vi "SLSC Separate Channels.vi"(8 "error in (no error)":errorcluster, 11 "Item Refs In":T1[](array[typedef]) format="%.0x") -> (0 "error out":errorcluster, 1 "Not Channels":T1[](array[typedef]) format="%.0x", 2 "Output Channels":T1[](array[typedef]) format="%.0x", 3 "Input Channels":T1[](array[typedef]) format="%.0x")   [LabVIEW 2020, in "SLSC EDS System Explorer.lvlib"]
uses:
  SLSC EDS System Explorer.lvlib
  <vilib>/NI VeriStand/Custom Device API/Custom Device Item Ref.ctl
  <vilib>/NI VeriStand/Custom Device API/Custom Device Channel Type.ctl
  <vilib>/NI VeriStand/Custom Device API/Custom Device API.lvlib
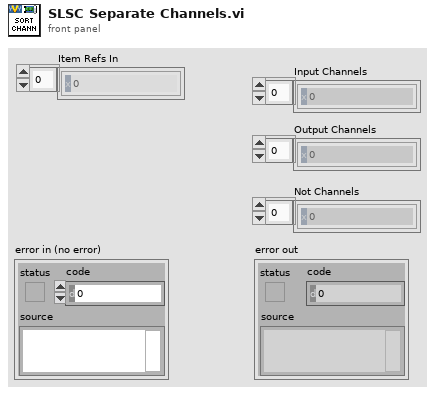
[diagram p1: front panel]
types:
  T1 = typedef "Custom Device API.lvlib/Custom Device Item Ref.ctl" = u64
  T2 = typedef "Custom Device API.lvlib/Custom Device Channel Type.ctl" = enum16{"Input", "Output"}
  T3 = typedef "Custom Device API.lvlib/Custom Device Channel.ctl" = cluster{"Type":T2, "Units":string, "Default Value":dbl, "Faultable":bool, "Scalable":bool}
  T4 = typedef "Custom Device API.lvlib/Custom Device Item Info.ctl" = cluster{"Name":string, "Is Channel":bool, "GUID":string, "Is Waveform":bool}
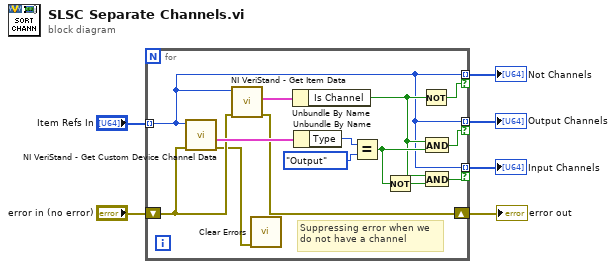
[diagram p0: block diagram]
diagram:
  n1 = for {
    tunnel: "Item Refs In" -> [w9] mode=indexing
    tunnel: [w9] -> w4 mode=indexing if=w13
    tunnel: [w9] -> w5 mode=indexing if=w14
    tunnel: [w9] -> w6 mode=indexing if=w11
    shift-right: [w10] -> w1
    shift-left: "error in (no error)" -> [w8]
    # "Suppressing error when we\ndo not have a channel"
    n2 = call <vilib>:"NI VeriStand - Get Custom Device Channel Data.vi"("error in (no error)"=w8, "Channel Ref in"=w9) -> ("error out"=w7:errorcluster, "Channel"=w20:T3)  [unwired: 4 in, 4 out]
    n3 = call <vilib>:"NI VeriStand - Get Item Data.vi"("error in (no error)"=w8, "Item Ref in"=w9) -> ("error out"=w10:errorcluster, "Item Info"=w19:T4)  [unwired: 6 in, 2 out]
    n4 = call <vilib>:"Clear Errors.vi"("error in (no error)"=w7) -> ()  [unwired: 5 in, 2 out]
    n5 = Unbundle By Name(w19) -> ("Is Channel"=w12:bool)
    n6 = Unbundle By Name(w20) -> ("Type"=w17:T2)
    n7 = Equal?(x=w17, y=Custom_Device_Channel_Type."Output" ("Type")) -> (x = y?=w15:bool)
    n8 = Not(x=w15) -> (.not. x?=w16:bool)
    n9 = Not(x=w12) -> (.not. x?=w11:bool)
    n10 = And(x=w12, y=w15) -> (x .and. y?=w13:bool)
    n11 = And(x=w12, y=w16) -> (x .and. y?=w14:bool)
  }
  "Not Channels" <- w6
  "Input Channels" <- w5
  "Output Channels" <- w4
  "error out" <- w1
